vi "Waveform Buffer Generation-Current.vi"(0 "task/channels in":refnum<k21>, 1 "Samples per Buffer":dbl=1000.0, 3 "Amplitude":dbl=2.0 format="%0.2p", 5 "Desired Frequency":dbl=1000.0 format="%.2f", 7 "Offset":dbl=0.01 format="%0.2p", 9 "Waveform Type":u16(ring) items=["Sine Wave", "Triangle Wave", "Square Wave", "Sawtooth Wave"], 11 "error in":errorcluster caption="error in (no error)", 12 "Cycles per Buffer":dbl=1.0 format="%.2f") -> (4 "task out":refnum<k21>, 6 "Waveform":waveform(dbl), 10 "Resulting Frequency":dbl format="%.2f", 14 "Resulting Sample Clock Rate":dbl format="%.2f", 15 "error out":errorcluster)   [LabVIEW 2022 SP3]
doc: "This subVI is used to create a Sine, Square, Triangle or Sawtooth Waveform. The inputs to this VI are the Waveform Type, which determines if the output waveform is a Sine, Square, Triangle, or Sawtooth Waveform, the amplitude, Desired Frequency, Samples per Buffer, and Cycles per Buffer. \n\nThe Desired Frequency, Samples per Buffer, and Cycles per Buffer are used to calculate the sample clock rate. The DAQmx Timing property node sets the sample clock rate for the device specified in the task/channels in control. \n\nThe actual, coerced, sample clock rate is returned and used as an input to the Basic Function Generator.vi. The Basic Function Generator returns a waveform of data with timing information.\n\nThe formula below was used to determine the sample clock rate:\n\nDesired Frequency=[(Cycles/Buffer)X(Sample Clock Rate)]/Samples per Buffer\n\nNote: The Block Diagram rearranges the variables to solve for Sample Clock Rate"
uses:
  <vilib>/measure/NI_MABase.lvlib
  <resource>/objmgr/daqmx.rc
panel:
  out "Samples/cycle":dbl format="%0.2f"
  out "Desired Sample Clock Rate":dbl format="%.2f"
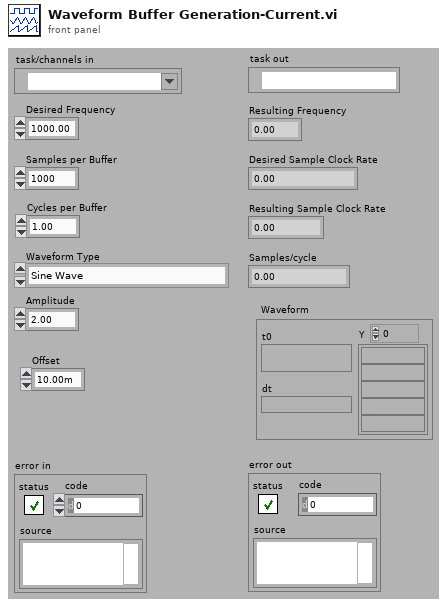
[diagram p1: front panel]
types:
  T1 = cluster{"SampClk.Rate":dbl, "Samples per Buffer":dbl}
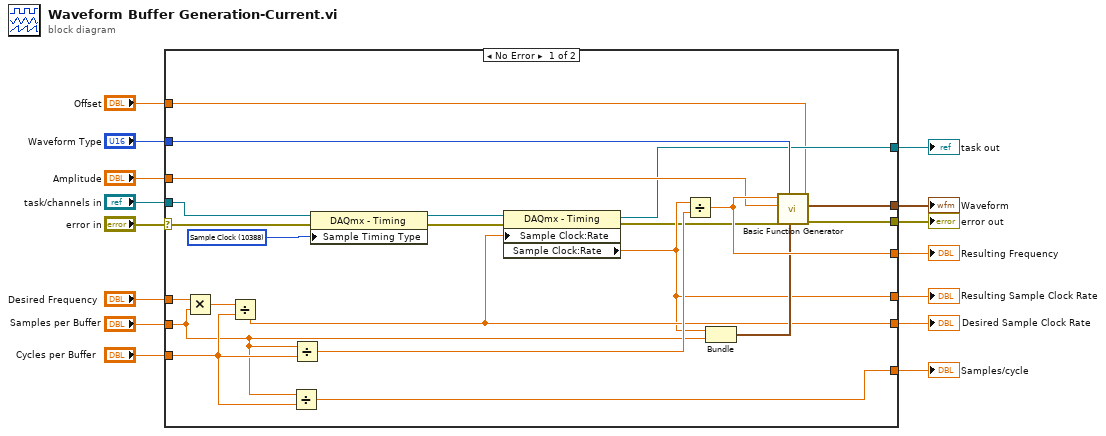
[diagram p0: block diagram]
diagram:
  n1 = case shown="No Error" "error in" {
    selector: "error in" -> [w16 w39]
    tunnel: [w37 _] -> w15
    tunnel: "Desired Frequency" -> [w36 _]
    tunnel: [w34 _] -> w13
    tunnel: [w32 _] -> w12
    tunnel: "Cycles per Buffer" -> [w31 _]
    tunnel: [w29 _] -> w10
    tunnel: "Waveform Type" -> [w28 _]
    tunnel: "Amplitude" -> [w27 _]
    tunnel: "Samples per Buffer" -> [w26 _]
    tunnel: [w25 w38] -> w6
    tunnel: [w24 _] -> w5
    tunnel: [w22 w39] -> w4
    tunnel: "task/channels in" -> [w18 w38]
    tunnel: "Offset" -> [w17 _]
    frame No Error {
      w19 = 10388 items=["Sample Clock"=10388, "Handshake"=10389, "Implicit"=10451, "On Demand"=10390, "Change Detection"=12504] ("SampTimingType")
      n2 = Multiply(x=w36, y=w26) -> (x*y=w33:dbl)
      n3 = Divide(x=w33, y=w31) -> (x/y=w29:dbl)
      n4 = Divide(x=w26, y=w31) -> (x/y=w32:dbl)
      n5 = Divide(x=w26, y=w31) -> (x/y=w30:dbl)
      n6 = property class="DAQmx - Timing"(reference=w18, error in=w16, "Sample Timing Type"=w19) -> (reference out=w21:refnum<k21>, error out=w20:errorcluster)
      n7 = property class="DAQmx - Timing"(reference=w21, error in=w20, "Sample Clock:Rate"=w29) -> (reference out=w25:refnum<k21>, error out=w23:errorcluster, "Sample Clock:Rate"=w24:dbl)
      n8 = Divide(x=w24, y=w30) -> (x/y=w37:dbl)
      n9 = Bundle("SampClk.Rate"=w24, "Samples per Buffer"=w26) -> (w35:T1)  [unwired: 1 in]
      n10 = call <vilib>:"Basic Function Generator.vi"("offset"=w17, "sampling info"=w35, "signal type"=w28, "error in (no error)"=w23, "amplitude"=w27, "frequency"=w37) -> ("error out"=w22:errorcluster, "signal out"=w34:waveform(dbl))  [unwired: 3 in, 1 out]
    }
    frame Error {
    }
  }
  "Resulting Sample Clock Rate" <- w5
  "Desired Sample Clock Rate" <- w10
  "Resulting Frequency" <- w15
  "Waveform" <- w13
  "Samples/cycle" <- w12
  "error out" <- w4
  "task out" <- w6
